vi "RIMAS Detector Read.vi"(7 "timeout (ms)":i32=3000, 8 "Error In":errorcluster, 11 "Detector Ref":refnum<k5>) -> (0 "Error Out":errorcluster, 1 "First String":string, 2 "data out":string, 3 "Detector Ref dup":refnum<k5>)   [LabVIEW 2022 SP3]
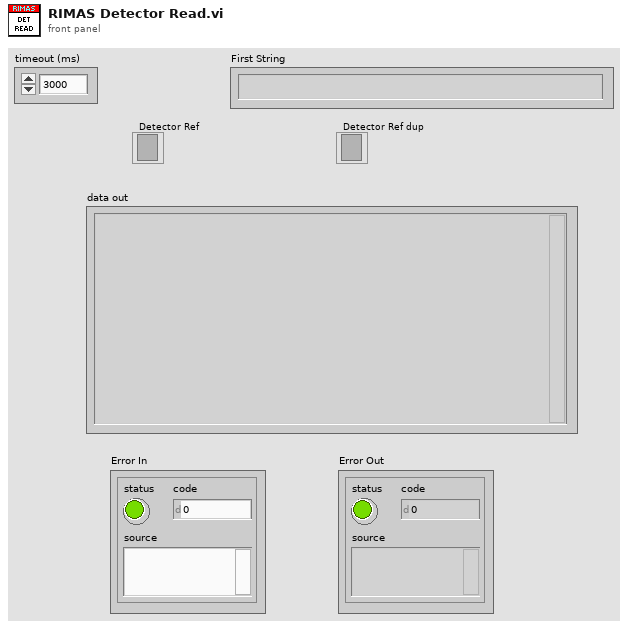
[diagram p1: front panel]
types:
  T1 = enum16{"Standard", "Buffered", "CRLF", "Immediate"}
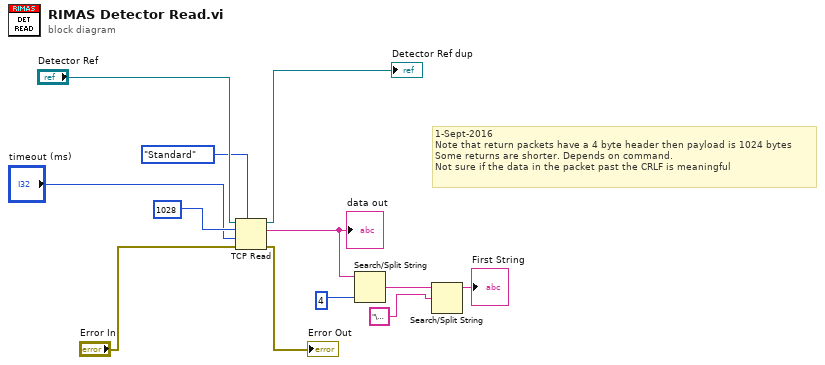
[diagram p0: block diagram]
diagram:
  # "1-Sept-2016\nNote that return packets have a 4 byte header then payload is 1024 bytes\nSome returns are shorter. Depends on command.\nNot sure if the data in the packet past the CRLF is meaningful"
  n1 = TCP Read(connection ID="Detector Ref", bytes to read=1028, error in (no error)="Error In", 7:T1."Standard" ("mode (standard)"), 9:"timeout (ms)") -> (connection ID out=→"Detector Ref dup":refnum<k5>, data out=w2:string, error out=→"Error Out":errorcluster)
  "data out" <- w2
  n2 = Search/Split String(string=w2, offset (0)=4) -> (match + rest of string=w3:string)  [unwired: 1 in, 2 out]
  n3 = Search/Split String(string=w3, search string/char (-)="\u0000") -> (substring before match=→"First String":string)  [unwired: 1 in, 2 out]
